vi "XML - Create XML file.vi"(8 "error in (no error)":errorcluster, 11 "CD Wizard - Internal Data":T1) -> (0 "error out":errorcluster, 3 "XML file path":path)   [LabVIEW 2015]
doc: "Create the XML file and alter the content of the file, so that it fits for the generated custom device."
uses:
  TypDef/CD Wizard - Internal data.ctl
  TypDef/CD Wizard - Execution Mode.ctl
  TypDef/CD Wizard - Extra Page Name and GUID.ctl
  TypDef/Create XML-file - States.ctl
  Constants/Constants TypDef/XML File.ctl
  Constants/Constants TypDef/CD System Explorer lvlib.ctl
  TypDef/Target Type.ctl
  Constants/XML File.vi
  Constants/CD System Explorer lvlib.vi
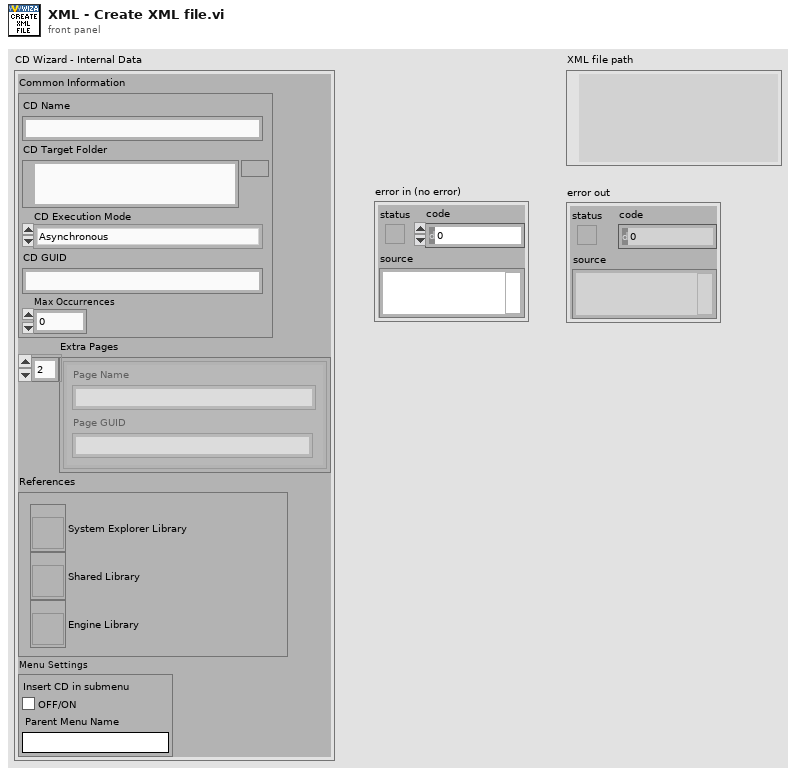
[diagram p1: front panel]
types:
  T1 = typedef "CD Wizard - Internal data.ctl" = cluster{"Common Information":cluster{"CD Name":string, "CD Target Folder":path, "CD Execution Mode":T2, "CD GUID":string, "Max Occurrences":u32}, "Extra Pages":T3[], "References":cluster{"System Explorer Library":refnum<vi>, "Shared Library":refnum<vi>, "Engine Library":refnum<vi>}, "Menu Settings":cluster{"Insert CD in submenu":bool, "Parent Menu Name":string}}
  T2 = typedef "CD Wizard - Execution Mode.ctl" = enum16{"Asynchronous", "Inline HW Interface", "Inline Model Interface", "Inline Timing and Sync", "Asynchronous Timing and Sync"}
  T3 = typedef "CD Wizard - Extra Page Name and GUID.ctl" = cluster{"Page Name":string, "Page GUID":string}
  T4 = typedef "Create XML-file - States.ctl" = enum16{"Initialize", "Copy XML template file", "Read XML file content", "Change CD -MenuName-", "Change CD -Name-", "Change CD -Type-", "Change CD -Occurrences-", "Change CD -MainPageGUID-", "Change CD -InitVIPath-", "Change CD -WindowsCustomDeviceVIPath-", "Change CD -WindowsCustomDeviceVIRTPath-", "Change CD -PharlapCustomDeviceVIPath-", "Change CD -PharlapCustomDeviceVIRTPath-", "Change CD -VxWorksCustomDeviceVIPath-", "Change CD -VxWorksCustomDeviceVIRTPath-", "Change CD -LinuxARMCustomDeviceVIPath-", "Change CD -LinuxARMCustomDeviceVIRTPath-", "Change CD -Linuxx64CustomDeviceVIPath-", "Change CD -Linuxx64CustomDeviceVIRTPath-", "Change CD -MainPageVIPath-", "Change CD -ExtraPages-", "Change CD -ActionVIOnCompile-", "Change CD -ExportConfigurationRTM-", "Write XML file content back", "Shutdown"}
  T5 = typedef "XML File.ctl" = enum16{"XMLTemplateFilePathAndName", "XMLTimingAndSyncFileName", "XMLCustomDeviceFileName"}
  T6 = typedef "CD System Explorer lvlib.ctl" = enum16{"LibraryFileName", "LibraryFolderName", "System Explorer.FolderName", "System Explorer.Dynamically Called.FolderName", "System Explorer.Dynamically Called.Extra Pages.FolderName", "System Explorer.Dynamically Called.Extra Pages.TemplatePathAndName", "System Explorer.Dynamically Called.Main Page.VIName", "System Explorer.Dynamically Called.Main Page.TemplatePathAndName", "System Explorer.Dynamically Called.Initialization VI.VIName", "System Explorer.Dynamically Called.Initialization VI.TemplatePathAndName", "System Explorer.SubVI.FolderName", "System Explorer.Types.FolderName", "System Explorer.ActionVIOnCompile.VIName", "System Explorer.ExportConfigRTM.VIName"}
  T7 = typedef "Target Type.ctl" = enum16{"Windows", "VxWorks", "Pharlap", "Linux 32 ARM", "Linux x64"}
  T8 = enum16{"open", "replace", "create", "open or create", "replace or create", "replace or create with confirmation"}
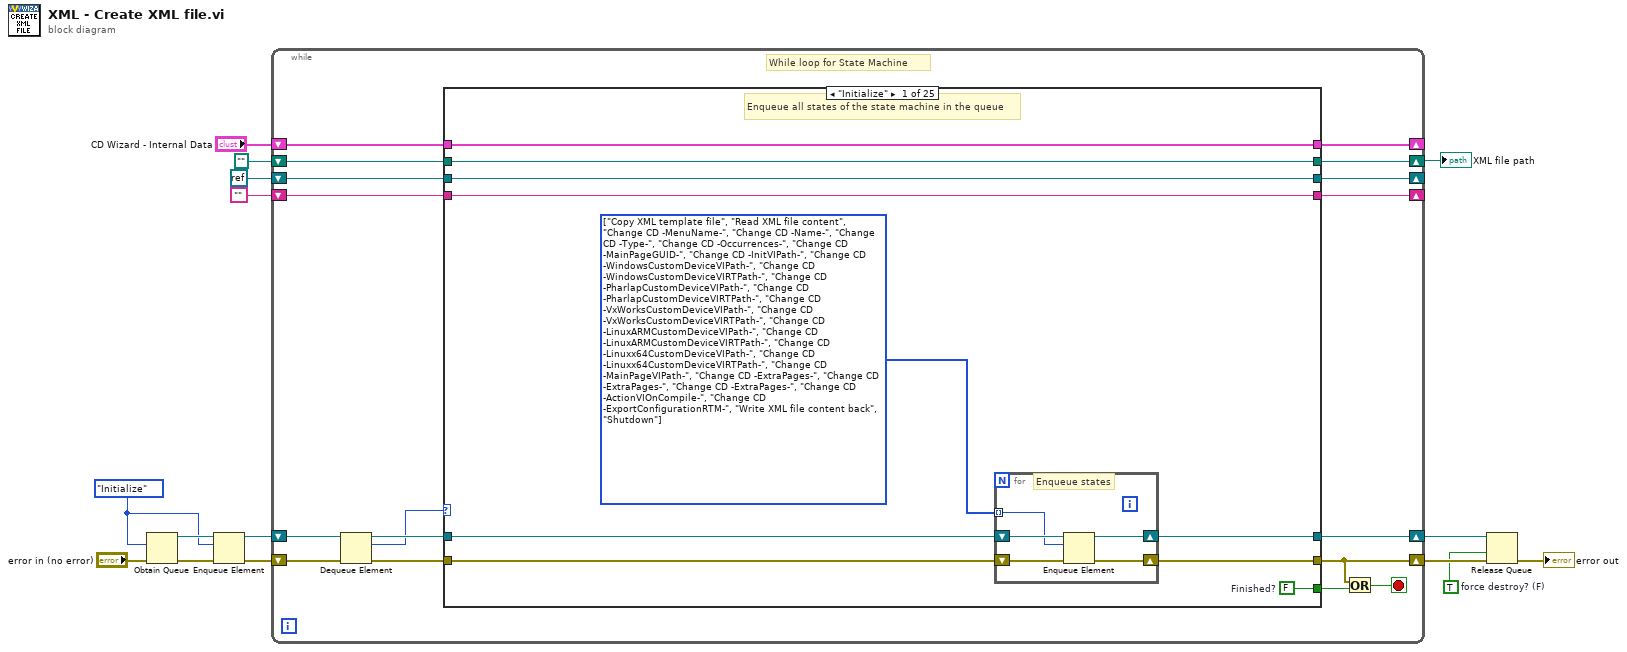
[diagram p0: block diagram]
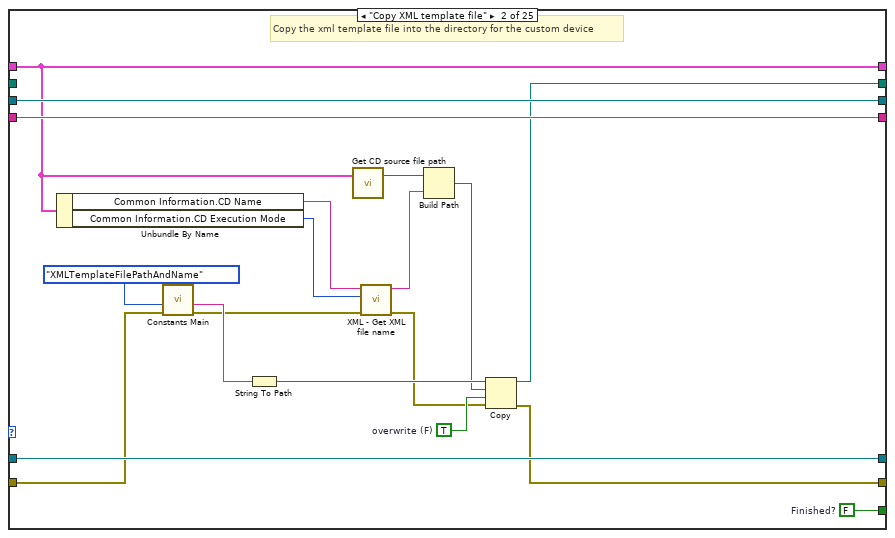
[diagram p2: hidden frame]
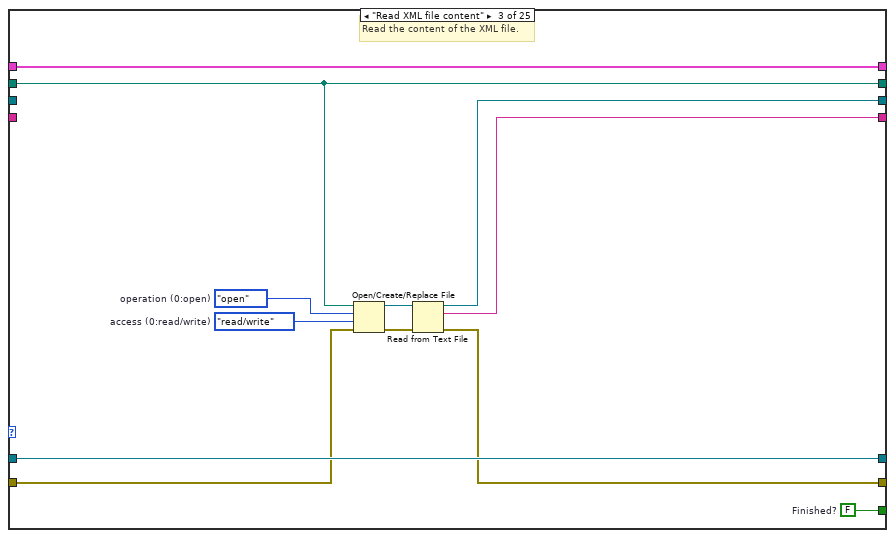
[diagram p3: hidden frame]
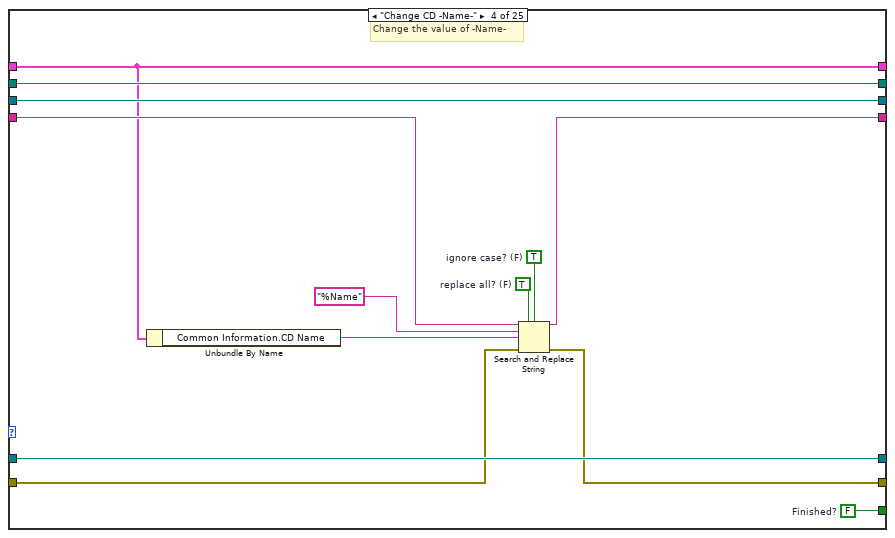
[diagram p4: hidden frame]
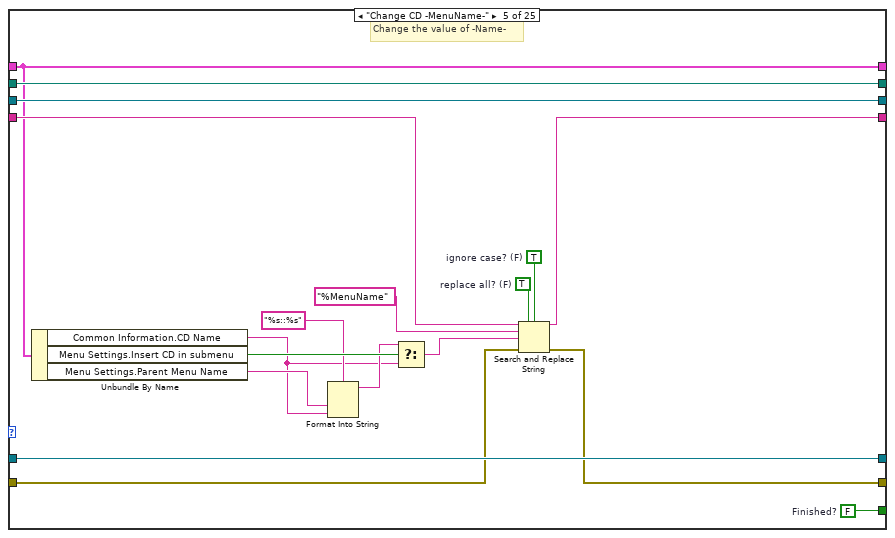
[diagram p5: hidden frame]
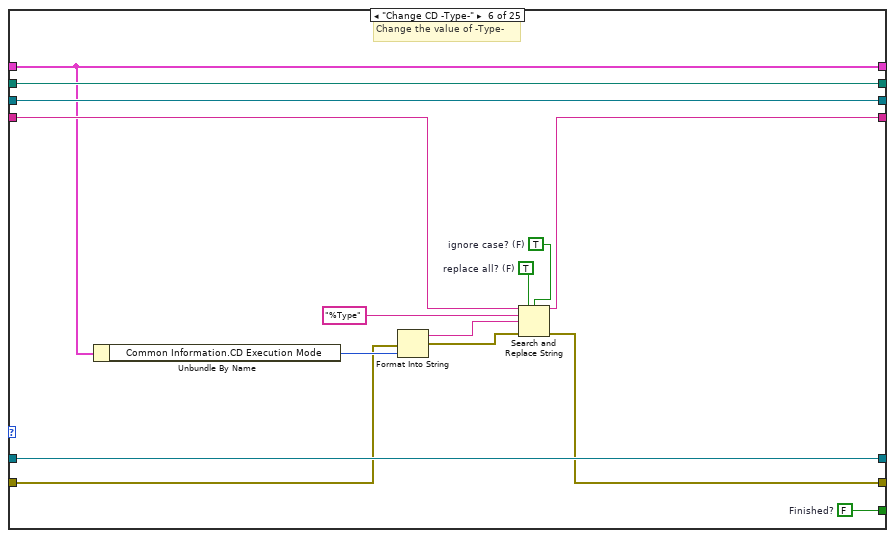
[diagram p6: hidden frame]
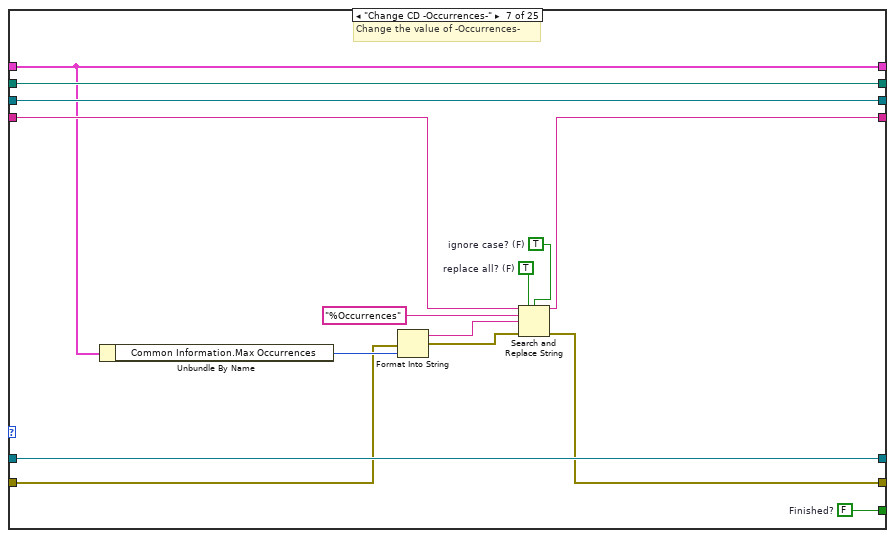
[diagram p7: hidden frame]
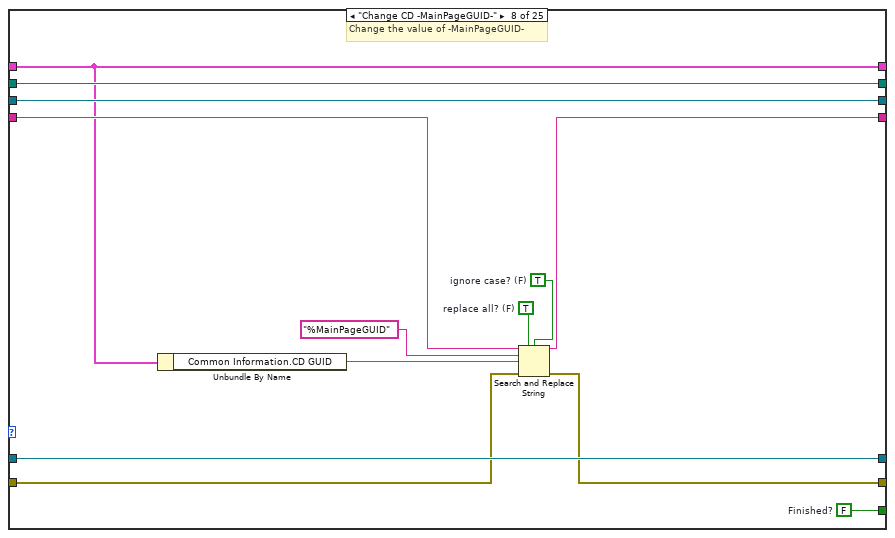
[diagram p8: hidden frame]
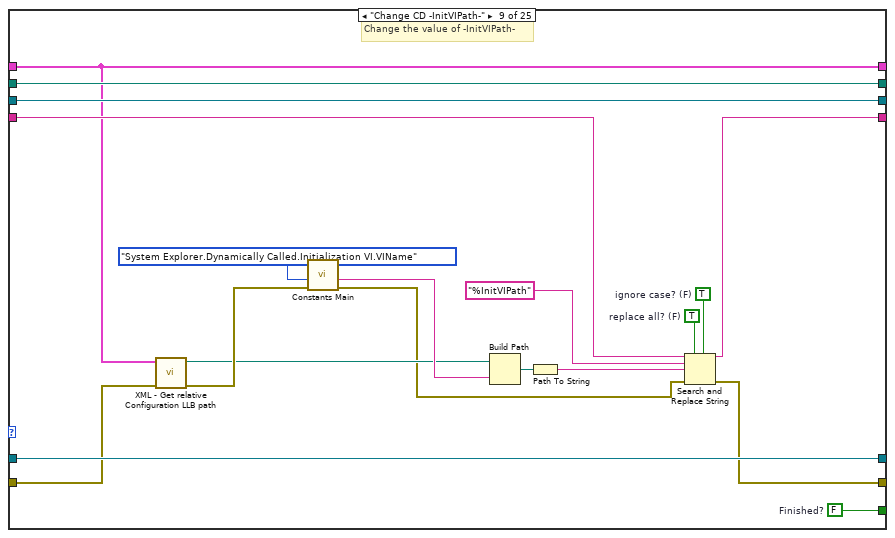
[diagram p9: hidden frame]
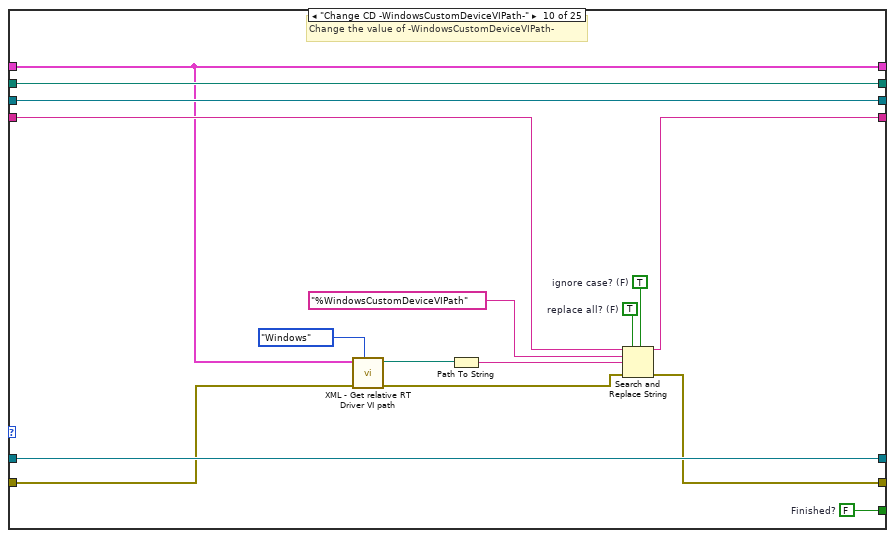
[diagram p10: hidden frame]
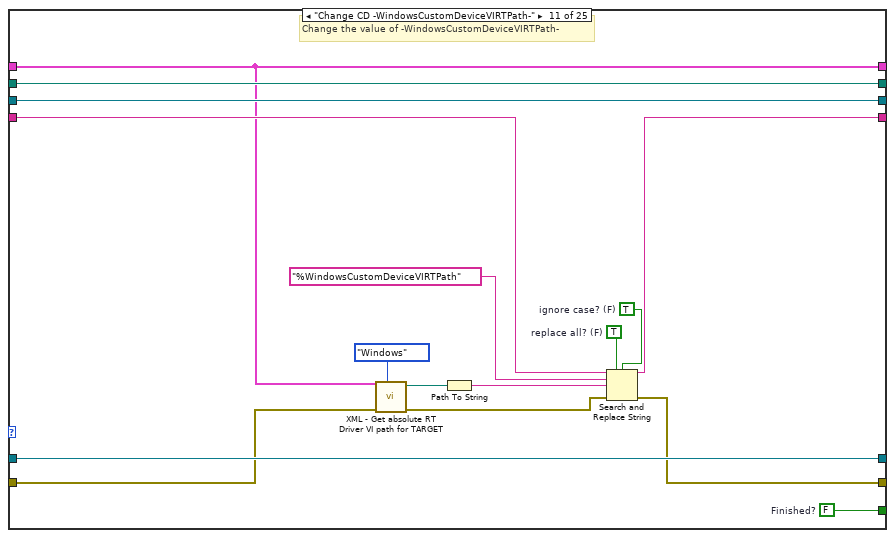
[diagram p11: hidden frame]
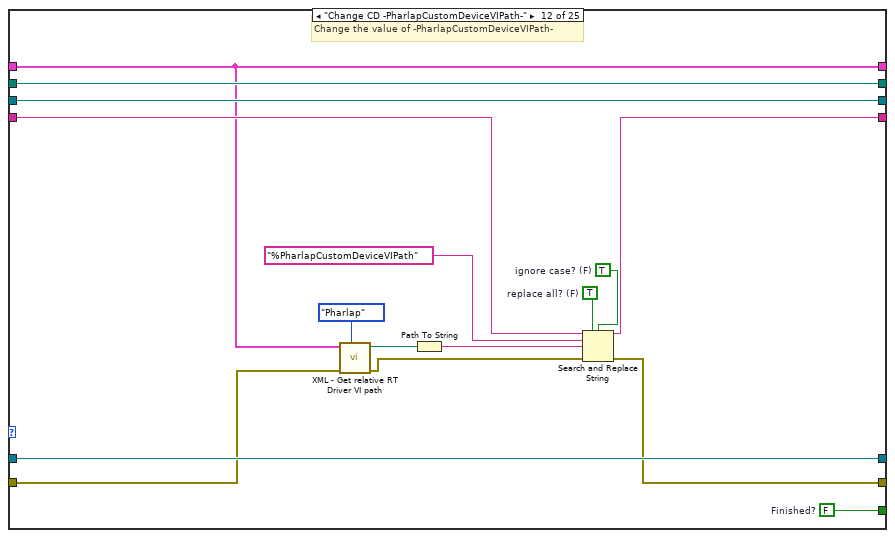
[diagram p12: hidden frame]
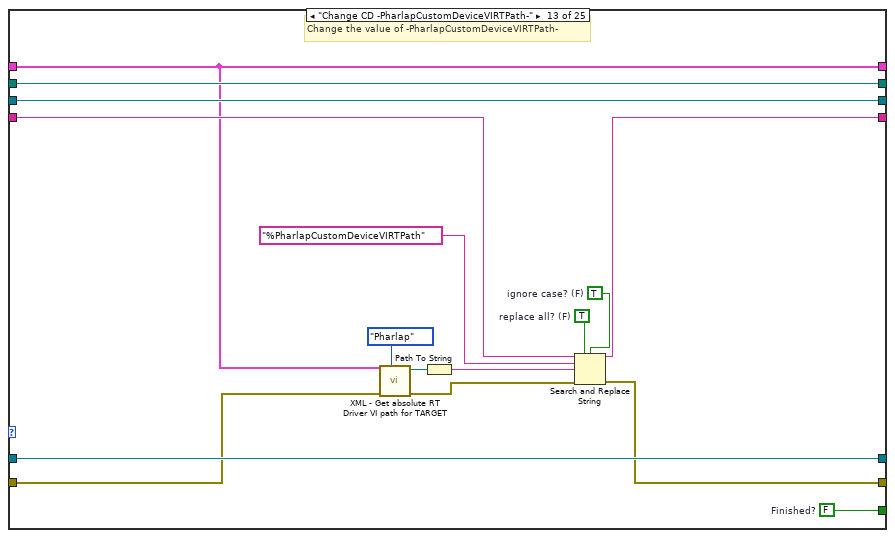
[diagram p13: hidden frame]
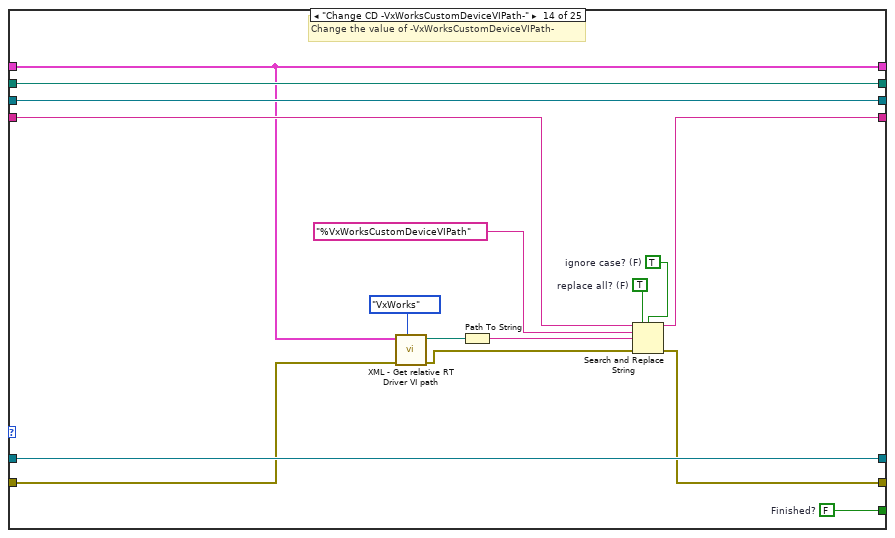
[diagram p14: hidden frame]
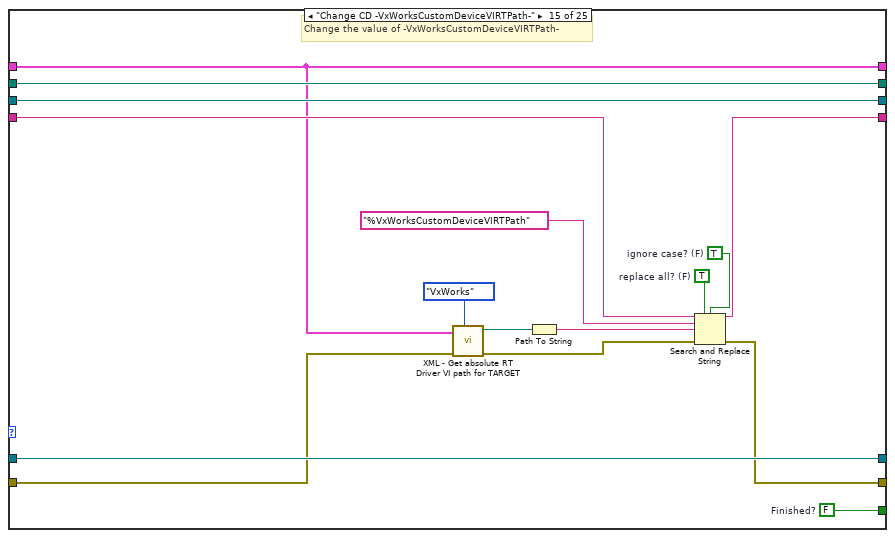
[diagram p15: hidden frame]
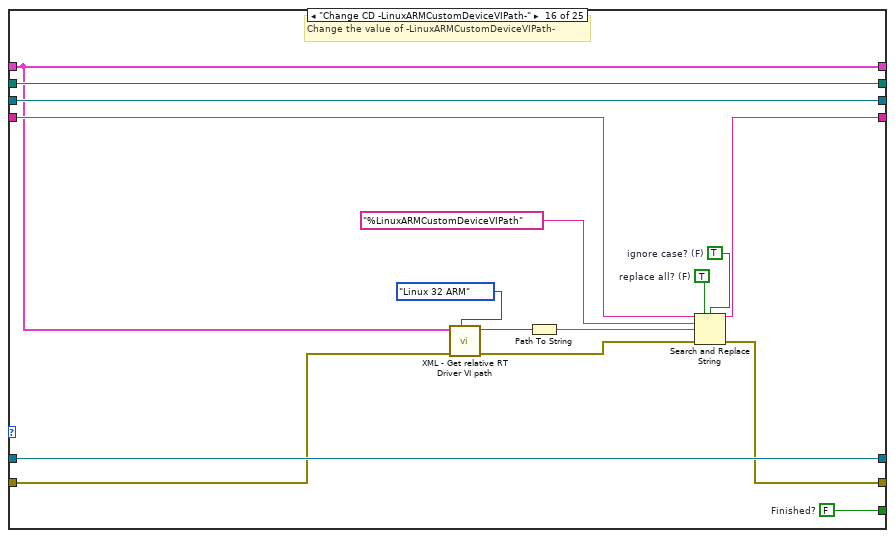
[diagram p16: hidden frame]
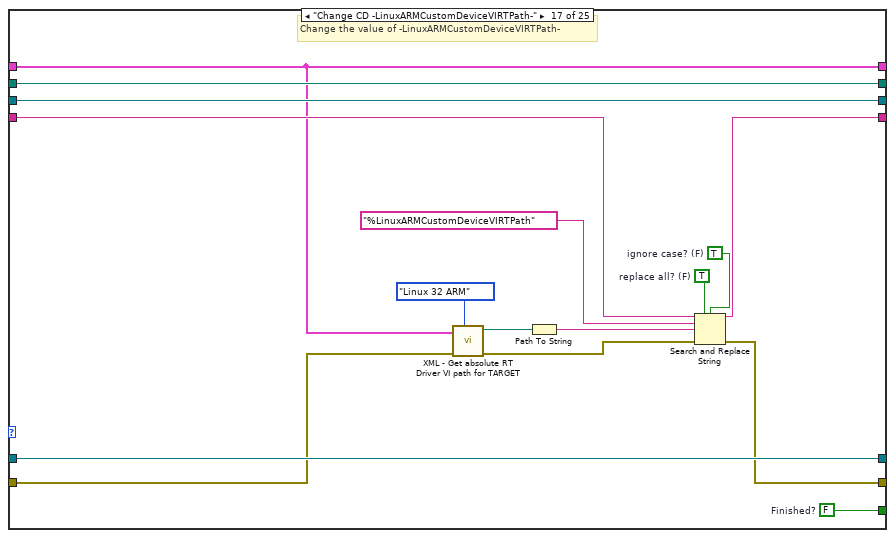
[diagram p17: hidden frame]
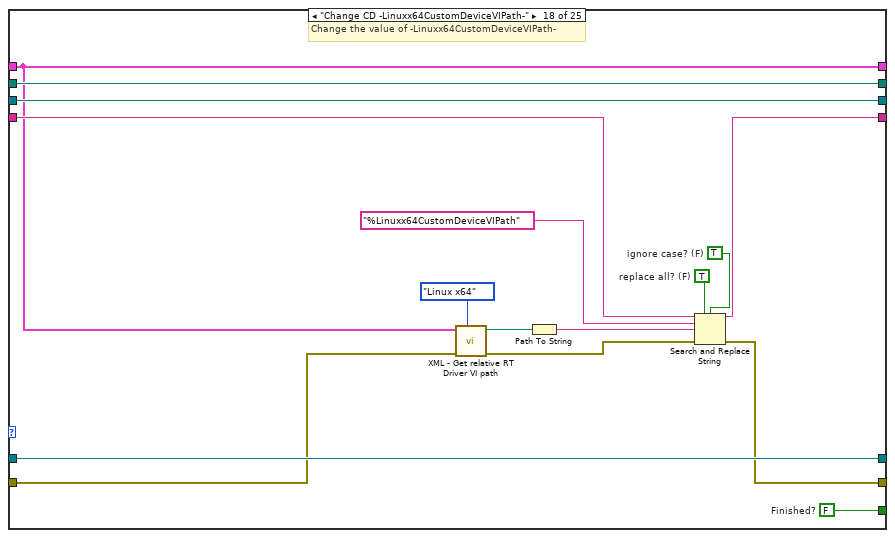
[diagram p18: hidden frame]
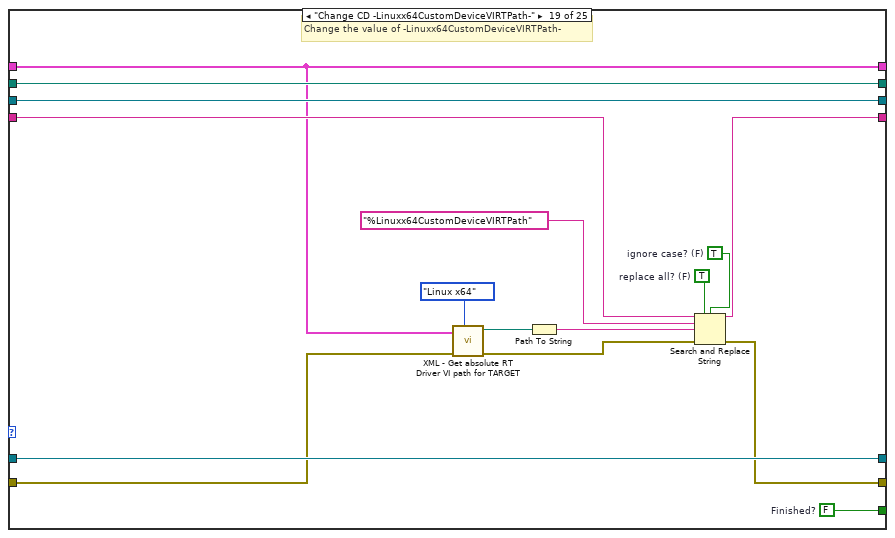
[diagram p19: hidden frame]
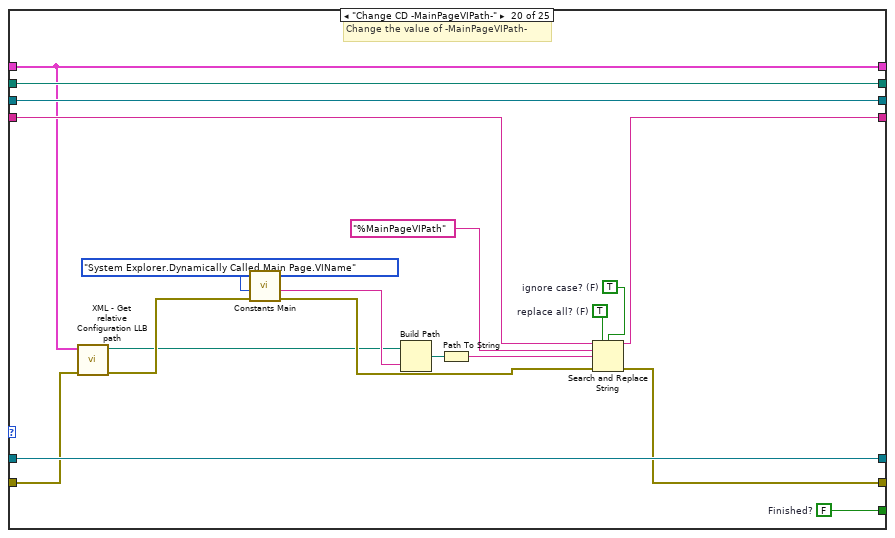
[diagram p20: hidden frame]
diagram:
  w8 = TRUE  # force destroy? (F)
  w5 = Create_XML-file_-_States."Initialize"
  n1 = Obtain Queue(element data type=w5, error in (no error)="error in (no error)") -> (queue out=w14:refnum<queue>, error out=w15:errorcluster)  [unwired: 3 in, 1 out]
  n2 = Enqueue Element(queue=w14, element=w5, error in (no error)=w15) -> (queue out=w13:refnum<queue>, error out=w12:errorcluster)  [unwired: 1 in, 1 out]
  n3 = while {
    shift-right: [w17] -> w9
    shift-left: w12 -> [w31]
    shift-right: [w26] -> _
    shift-left: "CD Wizard - Internal Data" -> [w27]
    shift-right: [w24] -> w1
    shift-left: path "" -> [w23]
    shift-right: [w22] -> _
    shift-left: refnum<k0> refnum -> [w21]
    shift-right: [w19] -> _
    shift-left: "" -> [w20]
    shift-right: [w25] -> w10
    shift-left: w13 -> [w32]
    stop <- w18 stop-if-true
    # "While loop for State Machine"
    n4 = Dequeue Element(queue=w32, error in (no error)=w31) -> (queue out=w29:refnum<queue>, element=w28:T4, error out=w30:errorcluster)  [unwired: 1 in, 1 out]
    n5 = case shown="\"Initialize\"" w28 {
      tunnel: w30 -> [w35 w59 w73 w84 w102 w112 w127 w142 w161 w174 w192 w206 w221 w238 w254 w270 w286 w302 w318 w334 w351 w372 w400 w413 w432]
      tunnel: w29 -> [w34 w64 w77 w91 w109 w124 w139 w152 w171 w187 w203 w219 w235 w251 w267 w283 w299 w315 w331 w350 w364 w383 w407 w424 w430]
      tunnel: [w36 w58 w71 w85 w103 w118 w133 w146 w165 w183 w198 w214 w230 w246 w262 w278 w294 w310 w326 w344 w358 w377 w384 w412 w432] -> w17
      tunnel: w27 -> [w42 w48 w78 w83 w101 w117 w132 w145 w160 w177 w191 w207 w223 w239 w255 w271 w287 w303 w319 w333 w356 w373 w401 w425 w431]
      tunnel: [w42 w48 w78 w83 w101 w117 w132 w145 w160 w177 w191 w207 w223 w239 w255 w271 w287 w303 w319 w333 w356 w373 w401 w425 w431] -> w26
      tunnel: [w37 w64 w77 w91 w109 w124 w139 w152 w171 w187 w203 w219 w235 w251 w267 w283 w299 w315 w331 w350 w364 w383 w407 w424 w430] -> w25
      tunnel: [w41 w57 w74 w90 w108 w123 w138 w151 w170 w186 w202 w218 w234 w250 w266 w282 w298 w314 w330 w349 w363 w382 w406 w423 w429] -> w24
      tunnel: w23 -> [w41 _ w74 w90 w108 w123 w138 w151 w170 w186 w202 w218 w234 w250 w266 w282 w298 w314 w330 w349 w363 w382 w406 w423 w429]
      tunnel: [w40 w66 w72 w89 w107 w122 w137 w150 w169 w185 w201 w217 w233 w249 w265 w281 w297 w313 w329 w348 w362 w381 w405 w408 w428] -> w22
      tunnel: w21 -> [w40 w66 _ w89 w107 w122 w137 w150 w169 w185 w201 w217 w233 w249 w265 w281 w297 w313 w329 w348 w362 w381 w405 w415 w428]
      tunnel: w20 -> [w39 w65 _ w87 w105 w120 w135 w148 w167 w179 w200 w216 w232 w248 w264 w280 w296 w312 w328 w346 w360 w379 w403 w414 w427]
      tunnel: [w39 w65 w70 w86 w104 w119 w134 w147 w166 w184 w199 w215 w231 w247 w263 w279 w295 w311 w327 w345 w359 w378 w388 w414 w427] -> w19
      tunnel: [w38 w55 w69 w80 w99 w111 w126 w141 w163 w181 w196 w212 w228 w244 w260 w276 w292 w308 w324 w342 w354 w375 w402 w411 w426] -> w16
      frame "Initialize" {
        w33 = T4[] [enum."Copy XML template file", enum."Read XML file content", enum."Change CD -MenuName-", enum."Change CD -Name-", enum."Change CD -Type-", enum."Change CD -Occurrences-", enum."Change CD -MainPageGUID-", enum."Change CD -InitVIPath-", enum."Change CD -WindowsCustomDeviceVIPath-", enum."Change CD -WindowsCustomDeviceVIRTPath-", enum."Change CD -PharlapCustomDeviceVIPath-", enum."Change CD -PharlapCustomDeviceVIRTPath-", enum."Change CD -VxWorksCustomDeviceVIPath-", enum."Change CD -VxWorksCustomDeviceVIRTPath-", enum."Change CD -LinuxARMCustomDeviceVIPath-", enum."Change CD -LinuxARMCustomDeviceVIRTPath-", enum."Change CD -Linuxx64CustomDeviceVIPath-", enum."Change CD -Linuxx64CustomDeviceVIRTPath-", enum."Change CD -MainPageVIPath-", enum."Change CD -ExtraPages-", enum."Change CD -ExtraPages-", enum."Change CD -ExtraPages-", enum."Change CD -ActionVIOnCompile-", enum."Change CD -ExportConfigurationRTM-", enum."Write XML file content back", enum."Shutdown"] items=["Initialize", "Copy XML template file", "Read XML file content", "Change CD -MenuName-", "Change CD -Name-", "Change CD -Type-", "Change CD -Occurrences-", "Change CD -MainPageGUID-", "Change CD -InitVIPath-", "Change CD -WindowsCustomDeviceVIPath-", "Change CD -WindowsCustomDeviceVIRTPath-", "Change CD -PharlapCustomDeviceVIPath-", "Change CD -PharlapCustomDeviceVIRTPath-", "Change CD -VxWorksCustomDeviceVIPath-", "Change CD -VxWorksCustomDeviceVIRTPath-", "Change CD -LinuxARMCustomDeviceVIPath-", "Change CD -LinuxARMCustomDeviceVIRTPath-", "Change CD -Linuxx64CustomDeviceVIPath-", "Change CD -Linuxx64CustomDeviceVIRTPath-", "Change CD -MainPageVIPath-", "Change CD -ExtraPages-", "Change CD -ActionVIOnCompile-", "Change CD -ExportConfigurationRTM-", "Write XML file content back", "Shutdown"]
        w38 = FALSE  # Finished?
        # "Enqueue all states of the state machine in the queue"
        n6 = for {
          shift-right: [w46] -> w37
          shift-left: w34 -> [w47]
          shift-right: [w45] -> w36
          shift-left: w35 -> [w44]
          tunnel: w33 -> [w43] mode=indexing
          # "Enqueue states"
          n7 = Enqueue Element(queue=w47, element=w43, error in (no error)=w44) -> (queue out=w46:refnum<queue>, error out=w45:errorcluster)  [unwired: 1 in, 1 out]
        }
      }
      frame "Copy XML template file" {
        w55 = FALSE  # Finished?
        w56 = TRUE  # overwrite (F)
        # "Copy the xml template file into the directory for the custom device"
        n8 = Unbundle By Name(w48) -> ("Common Information.CD Name"=w54:string, "Common Information.CD Execution Mode"=w53:T2)
        n9 = call-poly "Constants Main.vi"("error in (no error)"=w59, "Action"=XML_File."XMLTemplateFilePathAndName") -> ("error out"=w51:errorcluster, "Output"=w62:string)  [unwired: 8 in]
        n10 = String To Path(string=w62) -> (path=w61:path)
        n11 = call "Get CD source file path.vi"("CD Wizard - Internal Data"=w48) -> ("CD Source file path"=w49:path)  [unwired: 2 in]
        n12 = call "XML - Get XML file name.vi"("error in (no error)"=w51, "CD Execution Mode (Asynchronous)"=w53, "CD Name"=w54) -> ("error out"=w50:errorcluster, "XML file name"=w52:string)  [unwired: 7 in]
        n13 = Build Path(base path=w49, name or relative path=w52) -> (appended path=w60:path)
        n14 = Copy(8:w50, 9:w56, 10:w60, 11:w61) -> (0:w58:errorcluster, 3:w57:path)  [unwired: 2 out]
      }
      frame "Read XML file content" {
        w67 = T8."open"  # operation (0:open)
        w68 = enum16{"read/write", "read-only", "write-only"}."read/write"  # access (0:read/write)
        w69 = FALSE  # Finished?
        # "Read the content of the XML file."
        n15 = Open/Create/Replace File(file path (use dialog)=w74, error in=w73, operation (0:open)=w67, access (0:read/write)=w68) -> (refnum out=w76:refnum<file>, error out=w75:errorcluster)  [unwired: 3 out]
        n16 = Read from Text File(file (use dialog)=w76, error in=w75) -> (refnum out=w72:refnum<file>, text=w70:string, error out=w71:errorcluster)  [unwired: 3 out]
      }
      frame "Change CD -Name-" {
        w79 = TRUE  # ignore case? (F)
        w80 = FALSE  # Finished?
        w81 = TRUE  # replace all? (F)
        # "Change the value of -Name-"
        n17 = Unbundle By Name(w83) -> ("Common Information.CD Name"=w82:string)
        n18 = Search and Replace String(replace all?=w81, case sensitive?=w79, input string=w87, search string="%Name", replace string=w82, error in=w84) -> (result string=w86:string, error out=w85:errorcluster)  [unwired: 1 in, 3 out]
      }
      frame "Change CD -MenuName-" {
        w98 = TRUE  # ignore case? (F)
        w99 = FALSE  # Finished?
        w100 = TRUE  # replace all? (F)
        # "Change the value of -Name-"
        n19 = Unbundle By Name(w101) -> ("Common Information.CD Name"=w93:string, "Menu Settings.Insert CD in submenu"=w97:bool, "Menu Settings.Parent Menu Name"=w95:string)
        n20 = Format Into String(format string="%s::%s", w95, w93) -> (resulting string=w94:string)  [unwired: 2 in, 1 out]
        n21 = Select(t=w94, s=w97, f=w93) -> (s? t:f=w92:string)
        n22 = Search and Replace String(replace all?=w100, case sensitive?=w98, input string=w105, search string="%MenuName", replace string=w92, error in=w102) -> (result string=w104:string, error out=w103:errorcluster)  [unwired: 1 in, 3 out]
      }
      frame "Change CD -Type-" {
        w110 = TRUE  # ignore case? (F)
        w111 = FALSE  # Finished?
        w116 = TRUE  # replace all? (F)
        # "Change the value of -Type-"
        n23 = Unbundle By Name(w117) -> ("Common Information.CD Execution Mode"=w115:T2)
        n24 = Format Into String(error in=w112, w115) -> (resulting string=w114:string, error out=w113:errorcluster)  [unwired: 2 in]
        n25 = Search and Replace String(replace all?=w116, case sensitive?=w110, input string=w120, search string="%Type", replace string=w114, error in=w113) -> (result string=w119:string, error out=w118:errorcluster)  [unwired: 1 in, 3 out]
      }
      frame "Change CD -Occurrences-" {
        w125 = TRUE  # ignore case? (F)
        w126 = FALSE  # Finished?
        w131 = TRUE  # replace all? (F)
        # "Change the value of -Occurrences-"
        n26 = Unbundle By Name(w132) -> ("Common Information.Max Occurrences"=w130:u32)
        n27 = Format Into String(error in=w127, w130) -> (resulting string=w129:string, error out=w128:errorcluster)  [unwired: 2 in]
        n28 = Search and Replace String(replace all?=w131, case sensitive?=w125, input string=w135, search string="%Occurrences", replace string=w129, error in=w128) -> (result string=w134:string, error out=w133:errorcluster)  [unwired: 1 in, 3 out]
      }
      frame "Change CD -MainPageGUID-" {
        w140 = TRUE  # ignore case? (F)
        w141 = FALSE  # Finished?
        w144 = TRUE  # replace all? (F)
        # "Change the value of -MainPageGUID-"
        n29 = Unbundle By Name(w145) -> ("Common Information.CD GUID"=w143:string)
        n30 = Search and Replace String(replace all?=w144, case sensitive?=w140, input string=w148, search string="%MainPageGUID", replace string=w143, error in=w142) -> (result string=w147:string, error out=w146:errorcluster)  [unwired: 1 in, 3 out]
      }
      frame "Change CD -InitVIPath-" {
        w162 = TRUE  # ignore case? (F)
        w163 = FALSE  # Finished?
        w164 = TRUE  # replace all? (F)
        # "Change the value of -InitVIPath-"
        n31 = call "XML - Get relative Configuration LLB path.vi"("error in (no error)"=w161, "CD Wizard - Internal Data"=w160) -> ("error out"=w155:errorcluster, "Relative Configuration LLB path"=w154:path)  [unwired: 8 in]
        n32 = call-poly "Constants Main.vi"("error in (no error)"=w155, "Action"=CD_System_Explorer_lvlib."System Explorer.Dynamically Called.Initialization VI.VIName") -> ("error out"=w153:errorcluster, "Output"=w158:string)  [unwired: 8 in]
        n33 = Build Path(base path=w154, name or relative path=w158) -> (appended path=w156:path)
        n34 = Path To String(path=w156) -> (string=w159:string)
        n35 = Search and Replace String(replace all?=w164, case sensitive?=w162, input string=w167, search string="%InitVIPath", replace string=w159, error in=w153) -> (result string=w166:string, error out=w165:errorcluster)  [unwired: 1 in, 3 out]
      }
      frame "Change CD -WindowsCustomDeviceVIPath-" {
        w180 = TRUE  # ignore case? (F)
        w181 = FALSE  # Finished?
        w182 = TRUE  # replace all? (F)
        # "Change the value of -WindowsCustomDeviceVIPath-"
        n36 = call "XML - Get relative RT Driver VI path.vi"("Target Type (Windows)"=Target_Type."Windows", "error in (no error)"=w174, "CD Wizard - Internal Data"=w177) -> ("error out"=w172:errorcluster, "Relative RT Driver VI path"=w173:path)  [unwired: 7 in]
        n37 = Path To String(path=w173) -> (string=w176:string)
        n38 = Search and Replace String(replace all?=w182, case sensitive?=w180, input string=w179, search string="%WindowsCustomDeviceVIPath", replace string=w176, error in=w172) -> (result string=w184:string, error out=w183:errorcluster)  [unwired: 1 in, 3 out]
      }
      frame "Change CD -WindowsCustomDeviceVIRTPath-" {
        w195 = TRUE  # ignore case? (F)
        w196 = FALSE  # Finished?
        w197 = TRUE  # replace all? (F)
        # "Change the value of -WindowsCustomDeviceVIRTPath-"
        n39 = call "XML - Get absolute RT Driver VI path for TARGET.vi"("Target Type (Windows)"=Target_Type."Windows", "error in (no error)"=w192, "CD Wizard - Internal Data"=w191) -> ("error out"=w193:errorcluster, "Relative RT Driver TARGET path"=w188:path)  [unwired: 7 in]
        n40 = Path To String(path=w188) -> (string=w190:string)
        n41 = Search and Replace String(replace all?=w197, case sensitive?=w195, input string=w200, search string="%WindowsCustomDeviceVIRTPath", replace string=w190, error in=w193) -> (result string=w199:string, error out=w198:errorcluster)  [unwired: 1 in, 3 out]
      }
      frame "Change CD -PharlapCustomDeviceVIPath-" {
        w211 = TRUE  # ignore case? (F)
        w212 = FALSE  # Finished?
        w213 = TRUE  # replace all? (F)
        # "Change the value of -PharlapCustomDeviceVIPath-"
        n42 = call "XML - Get relative RT Driver VI path.vi"("Target Type (Windows)"=Target_Type."Pharlap", "error in (no error)"=w206, "CD Wizard - Internal Data"=w207) -> ("error out"=w209:errorcluster, "Relative RT Driver VI path"=w204:path)  [unwired: 7 in]
        n43 = Path To String(path=w204) -> (string=w205:string)
        n44 = Search and Replace String(replace all?=w213, case sensitive?=w211, input string=w216, search string="%PharlapCustomDeviceVIPath", replace string=w205, error in=w209) -> (result string=w215:string, error out=w214:errorcluster)  [unwired: 1 in, 3 out]
      }
      frame "Change CD -PharlapCustomDeviceVIRTPath-" {
        w227 = TRUE  # ignore case? (F)
        w228 = FALSE  # Finished?
        w229 = TRUE  # replace all? (F)
        # "Change the value of -PharlapCustomDeviceVIRTPath-"
        n45 = call "XML - Get absolute RT Driver VI path for TARGET.vi"("Target Type (Windows)"=Target_Type."Pharlap", "error in (no error)"=w221, "CD Wizard - Internal Data"=w223) -> ("error out"=w225:errorcluster, "Relative RT Driver TARGET path"=w220:path)  [unwired: 7 in]
        n46 = Path To String(path=w220) -> (string=w222:string)
        n47 = Search and Replace String(replace all?=w229, case sensitive?=w227, input string=w232, search string="%PharlapCustomDeviceVIRTPath", replace string=w222, error in=w225) -> (result string=w231:string, error out=w230:errorcluster)  [unwired: 1 in, 3 out]
      }
      frame "Change CD -VxWorksCustomDeviceVIPath-" {
        w243 = TRUE  # ignore case? (F)
        w244 = FALSE  # Finished?
        w245 = TRUE  # replace all? (F)
        # "Change the value of -VxWorksCustomDeviceVIPath-"
        n48 = call "XML - Get relative RT Driver VI path.vi"("Target Type (Windows)"=Target_Type."VxWorks", "error in (no error)"=w238, "CD Wizard - Internal Data"=w239) -> ("error out"=w241:errorcluster, "Relative RT Driver VI path"=w236:path)  [unwired: 7 in]
        n49 = Path To String(path=w236) -> (string=w237:string)
        n50 = Search and Replace String(replace all?=w245, case sensitive?=w243, input string=w248, search string="%VxWorksCustomDeviceVIPath", replace string=w237, error in=w241) -> (result string=w247:string, error out=w246:errorcluster)  [unwired: 1 in, 3 out]
      }
      frame "Change CD -VxWorksCustomDeviceVIRTPath-" {
        w259 = TRUE  # ignore case? (F)
        w260 = FALSE  # Finished?
        w261 = TRUE  # replace all? (F)
        # "Change the value of -VxWorksCustomDeviceVIRTPath-"
        n51 = call "XML - Get absolute RT Driver VI path for TARGET.vi"("Target Type (Windows)"=Target_Type."VxWorks", "error in (no error)"=w254, "CD Wizard - Internal Data"=w255) -> ("error out"=w257:errorcluster, "Relative RT Driver TARGET path"=w252:path)  [unwired: 7 in]
        n52 = Path To String(path=w252) -> (string=w253:string)
        n53 = Search and Replace String(replace all?=w261, case sensitive?=w259, input string=w264, search string="%VxWorksCustomDeviceVIRTPath", replace string=w253, error in=w257) -> (result string=w263:string, error out=w262:errorcluster)  [unwired: 1 in, 3 out]
      }
      frame "Change CD -LinuxARMCustomDeviceVIPath-" {
        w275 = TRUE  # ignore case? (F)
        w276 = FALSE  # Finished?
        w277 = TRUE  # replace all? (F)
        # "Change the value of -LinuxARMCustomDeviceVIPath-"
        n54 = call "XML - Get relative RT Driver VI path.vi"("Target Type (Windows)"=Target_Type."Linux 32 ARM", "error in (no error)"=w270, "CD Wizard - Internal Data"=w271) -> ("error out"=w268:errorcluster, "Relative RT Driver VI path"=w269:path)  [unwired: 7 in]
        n55 = Path To String(path=w269) -> (string=w273:string)
        n56 = Search and Replace String(replace all?=w277, case sensitive?=w275, input string=w280, search string="%LinuxARMCustomDeviceVIPath", replace string=w273, error in=w268) -> (result string=w279:string, error out=w278:errorcluster)  [unwired: 1 in, 3 out]
      }
      frame "Change CD -LinuxARMCustomDeviceVIRTPath-" {
        w291 = TRUE  # ignore case? (F)
        w292 = FALSE  # Finished?
        w293 = TRUE  # replace all? (F)
        # "Change the value of -LinuxARMCustomDeviceVIRTPath-"
        n57 = call "XML - Get absolute RT Driver VI path for TARGET.vi"("Target Type (Windows)"=Target_Type."Linux 32 ARM", "error in (no error)"=w286, "CD Wizard - Internal Data"=w287) -> ("error out"=w289:errorcluster, "Relative RT Driver TARGET path"=w284:path)  [unwired: 7 in]
        n58 = Path To String(path=w284) -> (string=w285:string)
        n59 = Search and Replace String(replace all?=w293, case sensitive?=w291, input string=w296, search string="%LinuxARMCustomDeviceVIRTPath", replace string=w285, error in=w289) -> (result string=w295:string, error out=w294:errorcluster)  [unwired: 1 in, 3 out]
      }
      frame "Change CD -Linuxx64CustomDeviceVIPath-" {
        w307 = TRUE  # ignore case? (F)
        w308 = FALSE  # Finished?
        w309 = TRUE  # replace all? (F)
        # "Change the value of -Linuxx64CustomDeviceVIPath-"
        n60 = call "XML - Get relative RT Driver VI path.vi"("Target Type (Windows)"=Target_Type."Linux x64", "error in (no error)"=w302, "CD Wizard - Internal Data"=w303) -> ("error out"=w300:errorcluster, "Relative RT Driver VI path"=w301:path)  [unwired: 7 in]
        n61 = Path To String(path=w301) -> (string=w305:string)
        n62 = Search and Replace String(replace all?=w309, case sensitive?=w307, input string=w312, search string="%Linuxx64CustomDeviceVIPath", replace string=w305, error in=w300) -> (result string=w311:string, error out=w310:errorcluster)  [unwired: 1 in, 3 out]
      }
      frame "Change CD -Linuxx64CustomDeviceVIRTPath-" {
        w323 = TRUE  # ignore case? (F)
        w324 = FALSE  # Finished?
        w325 = TRUE  # replace all? (F)
        # "Change the value of -Linuxx64CustomDeviceVIRTPath-"
        n63 = call "XML - Get absolute RT Driver VI path for TARGET.vi"("Target Type (Windows)"=Target_Type."Linux x64", "error in (no error)"=w318, "CD Wizard - Internal Data"=w319) -> ("error out"=w321:errorcluster, "Relative RT Driver TARGET path"=w316:path)  [unwired: 7 in]
        n64 = Path To String(path=w316) -> (string=w317:string)
        n65 = Search and Replace String(replace all?=w325, case sensitive?=w323, input string=w328, search string="%Linuxx64CustomDeviceVIRTPath", replace string=w317, error in=w321) -> (result string=w327:string, error out=w326:errorcluster)  [unwired: 1 in, 3 out]
      }
      frame "Change CD -MainPageVIPath-" {
        w341 = TRUE  # ignore case? (F)
        w342 = FALSE  # Finished?
        w343 = TRUE  # replace all? (F)
        # "Change the value of -MainPageVIPath-"
        n66 = call "XML - Get relative Configuration LLB path.vi"("error in (no error)"=w334, "CD Wizard - Internal Data"=w333) -> ("error out"=w337:errorcluster, "Relative Configuration LLB path"=w332:path)  [unwired: 8 in]
        n67 = call-poly "Constants Main.vi"("error in (no error)"=w337, "Action"=CD_System_Explorer_lvlib."System Explorer.Dynamically Called.Main Page.VIName") -> ("error out"=w335:errorcluster, "Output"=w340:string)  [unwired: 8 in]
        n68 = Build Path(base path=w332, name or relative path=w340) -> (appended path=w338:path)
        n69 = Path To String(path=w338) -> (string=w336:string)
        n70 = Search and Replace String(replace all?=w343, case sensitive?=w341, input string=w346, search string="%MainPageVIPath", replace string=w336, error in=w335) -> (result string=w345:string, error out=w344:errorcluster)  [unwired: 1 in, 3 out]
      }
      frame "Change CD -ExtraPages-" {
        w353 = TRUE  # ignore case? (F)
        w354 = FALSE  # Finished?
        w357 = TRUE  # replace all? (F)
        # "Change the value of -ExtraPages-"
        n71 = call "XML - Get extra pages XML string.vi"("error in (no error)"=w351, "CD Wizard - Internal Data"=w356) -> ("error out"=w352:errorcluster, "Extra Pages XML string"=w355:string)  [unwired: 8 in]
        n72 = Search and Replace String(replace all?=w357, case sensitive?=w353, input string=w360, search string="%ExtraPages", replace string=w355, error in=w352) -> (result string=w359:string, error out=w358:errorcluster)  [unwired: 1 in, 3 out]
      }
      frame "Change CD -ActionVIOnCompile-" {
        w374 = TRUE  # ignore case? (F)
        w375 = FALSE  # Finished?
        w376 = TRUE  # replace all? (F)
        # "Change the value of -ActionVIOnCompile-"
        n73 = call "XML - Get relative Configuration LLB path.vi"("error in (no error)"=w372, "CD Wizard - Internal Data"=w373) -> ("error out"=w367:errorcluster, "Relative Configuration LLB path"=w371:path)  [unwired: 8 in]
        n74 = call-poly "Constants Main.vi"("error in (no error)"=w367, "Action"=CD_System_Explorer_lvlib."System Explorer.ActionVIOnCompile.VIName") -> ("error out"=w366:errorcluster, "Output"=w365:string)  [unwired: 8 in]
        n75 = Build Path(base path=w371, name or relative path=w365) -> (appended path=w370:path)
        n76 = Path To String(path=w370) -> (string=w369:string)
        n77 = Search and Replace String(replace all?=w376, case sensitive?=w374, input string=w379, search string="%ActionVICompilePath", replace string=w369, error in=w366) -> (result string=w378:string, error out=w377:errorcluster)  [unwired: 1 in, 3 out]
      }
      frame "Change CD -ExportConfigurationRTM-" {
        w391 = TRUE  # ignore case? (F)
        w402 = FALSE  # Finished?
        w390 = TRUE  # replace all? (F)
        # "Change the value of -ExportConfigurationRTM-"
        n78 = call "XML - Get relative Configuration LLB path.vi"("error in (no error)"=w400, "CD Wizard - Internal Data"=w401) -> ("error out"=w395:errorcluster, "Relative Configuration LLB path"=w399:path)  [unwired: 8 in]
        n79 = call-poly "Constants Main.vi"("error in (no error)"=w395, "Action"=CD_System_Explorer_lvlib."System Explorer.ExportConfigRTM.VIName") -> ("error out"=w394:errorcluster, "Output"=w393:string)  [unwired: 8 in]
        n80 = Build Path(base path=w399, name or relative path=w393) -> (appended path=w398:path)
        n81 = Path To String(path=w398) -> (string=w397:string)
        n82 = Search and Replace String(replace all?=w390, case sensitive?=w391, input string=w403, search string="%ExportConfigurationRTMPath", replace string=w397, error in=w394) -> (result string=w389:string, error out=w387:errorcluster)  [unwired: 1 in, 3 out]
        n83 = call "Create GUID.vi"("error in (no error)"=w387) -> ("error out"=w385:errorcluster, "Generated GUID"=w386:string)  [unwired: 9 in]
        n84 = Search and Replace String(replace all?=w390, case sensitive?=w391, input string=w389, search string="%ExportConfigurationGUID", replace string=w386, error in=w385) -> (result string=w388:string, error out=w384:errorcluster)  [unwired: 1 in, 3 out]
      }
      frame "Write XML file content back" {
        w408 = refnum<file> refnum  # refnum out
        w411 = FALSE  # Finished?
        w416 = enum16{"start", "end", "current"}."start"  # from (0:start)
        # "Write the modified file content back to the XML file"
        n85 = String Length(string=w414) -> (length=w410:i32)
        n86 = Set File Position(refnum=w415, from (0:start)=w416, error in=w413) -> (refnum out=w417:refnum<file>, error out=w418:errorcluster)  [unwired: 1 out]
        n87 = To Quad Integer(1:w410) -> (0:w409:i64)
        n88 = Set File Size(4:w418, 6:w409, 7:w417) -> (0:w420:errorcluster, 3:w419:refnum<file>)
        n89 = Write to Text File(file (use dialog)=w419, text=w414, error in=w420) -> (refnum out=w422:refnum<file>, error out=w421:errorcluster)  [unwired: 2 out]
        n90 = Close File(refnum=w422, error in=w421) -> (error out=w412:errorcluster)  [unwired: 1 out]
      }
      frame "Shutdown" {
        w426 = TRUE  # Finished?
        # "Shut down the state machine"
      }
    }
    n91 = Or(x=w17, y=w16) -> (x .or. y?=w18:bool)
  }
  "XML file path" <- w1
  n92 = Release Queue(queue=w10, force destroy? (F)=w8, error in (no error)=w9) -> (error out=→"error out":errorcluster)  [unwired: 2 out]
